vi "doc_get_subtable_keys.vi"(7 "subtables":string[](array[string]), 8 "error in (no error)":errorcluster, 10 "Doc in":refnum<class "Doc.lvclass">) -> (0 "error out":errorcluster, 1 "keys":string[](array[string]), 2 "Doc out":refnum<class "Doc.lvclass">, 4 "found?":bool)   [LabVIEW 2020, in "toml.lvclass"]
uses:
  toml.lvclass
  Doc/Doc.lvclass
  toml.lvclass/toml.ctl
  Table/Table.lvclass
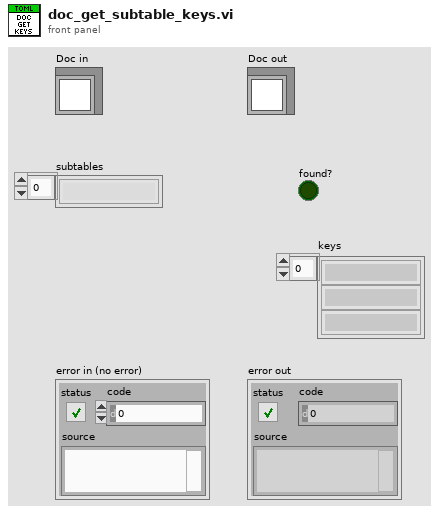
[diagram p1: front panel]
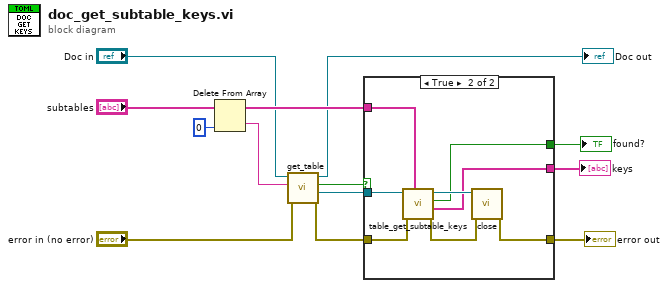
[diagram p0: block diagram]
diagram:
  n1 = Delete From Array(array="subtables", index=0) -> (deleted portion=w11:string, array with subset deleted=w13:string[])  [unwired: 1 in]
  n2 = call "get_table.vi"("error in (no error)"="error in (no error)", "table_name"=w11, "Doc in"="Doc in") -> ("error out"=w10:errorcluster, "Table"=w2:refnum<class "Table.lvclass">, "found?"=w1:bool, "Doc out"=→"Doc out":refnum<class "Doc.lvclass">)  [unwired: 5 in]
  n3 = case shown="True" w1 {
    selector: w1 -> [w15 _]
    tunnel: w13 -> [_ w23]
    tunnel: w10 -> [w14 w22]
    tunnel: [w14 w19] -> w5
    tunnel: [w15 w18] -> w4
    tunnel: [_ w17] -> w3
    tunnel: w2 -> [_ w16]
    frame False {
    }
    frame True {
      n4 = call "table_get_subtable_keys.vi"("subtables"=w23, "error in (no error)"=w22, "Table in"=w16) -> ("error out"=w20:errorcluster, "keys"=w17:string[], "found subtable?"=w18:bool, "Table out"=w21:refnum<class "Table.lvclass">)  [unwired: 5 in]
      n5 = call "close.vi"("error in (no error)"=w20, "Table in"=w21) -> ("error out"=w19:errorcluster)  [unwired: 9 in]
    }
  }
  "error out" <- w5
  "keys" <- w3
  "found?" <- w4
